vi "GA Set Gear Event.vi"(7 "startPara1":dbl, 8 "error in (no error)":errorcluster caption="错误输入（无错误）", 9 "startPara0":dbl, 10 "nEvent":i16, 11 "nAxisNum":i16) -> (0 "error out":errorcluster caption="错误输出", 3 "function return":i32)   [LabVIEW 2015, in "GAS.lvlib"]
doc: "extern \"C\" __declspec(dllimport) int GA_SetGearEvent(short nAxisNum,short nEvent,double startPara0,double startPara1);"
uses:
  <userlib>/BP_GAS/GAS.lvlib
  <userlib>/BP_GAS/GAS.dll
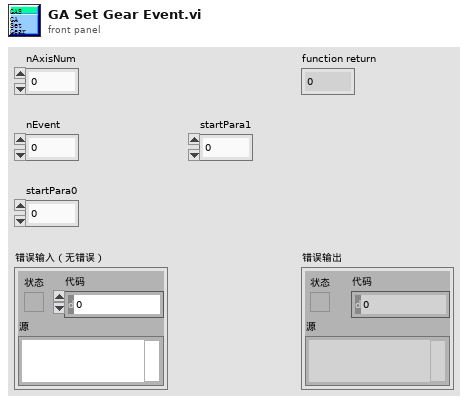
[diagram p1: front panel]
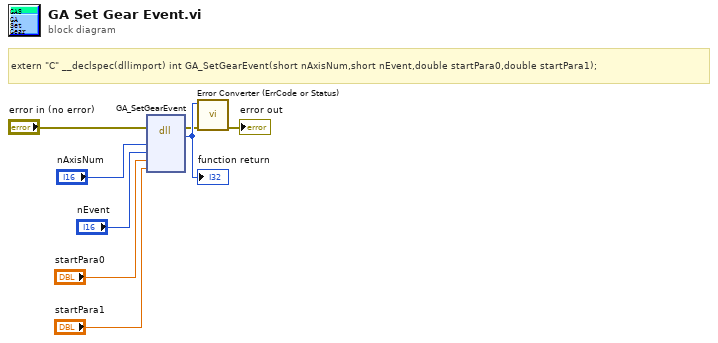
[diagram p0: block diagram]
diagram:
  # "extern \"C\" __declspec(dllimport) int GA_SetGearEvent(short nAxisNum,short nEvent,double startPara0,double startPara1);"
  n1 = dll-call lib="E:/Program Files (x86)/National Instruments/LabVIEW 2015/user.lib/BP_GAS/GAS.*" fn="GA_SetGearEvent"(error in="error in (no error)", "nAxisNum"="nAxisNum", "nEvent"="nEvent", "startPara0"="startPara0", "startPara1"="startPara1") -> (error out=w2:errorcluster, w8:i32)  [unwired: 6 in, 1 out]
  "function return" <- w8
  n2 = call "Error Converter (ErrCode or Status).vi"("error in (no error)"=w2, "error code"=w8) -> ("error out"=→"error out":errorcluster)  [unwired: 9 in]
